vi "nVI.vi"() -> ()   [LabVIEW 2021]
panel:
  out "String 2":string
  out "Boolean 2":bool
  out "Numeric 2":dbl
  in  "String":string
  in  "Numeric":dbl
  in  "Boolean":bool
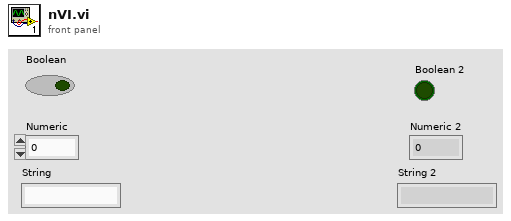
[diagram p1: front panel]
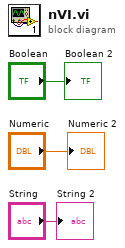
[diagram p0: block diagram]
diagram:
  "Numeric 2" <- "Numeric"
  "Boolean 2" <- "Boolean"
  "String 2" <- "String"
